vi "I32Notifier Wait2Get.vi"(8 "error in (no error)":errorcluster, 9 "timeout in ms (-1)":i32, 11 "I32Notifier in":refnum<class "I32Notifier.lvclass">) -> (0 "error out":errorcluster, 1 "timed out?":bool, 2 "LastValue":i32, 3 "I32Notifier out":refnum<class "I32Notifier.lvclass">)   [LabVIEW 2018, in "I32Notifier.lvclass"]
uses:
  I32Notifier.lvclass
  I32Notifier.lvclass/I32Notifier.ctl
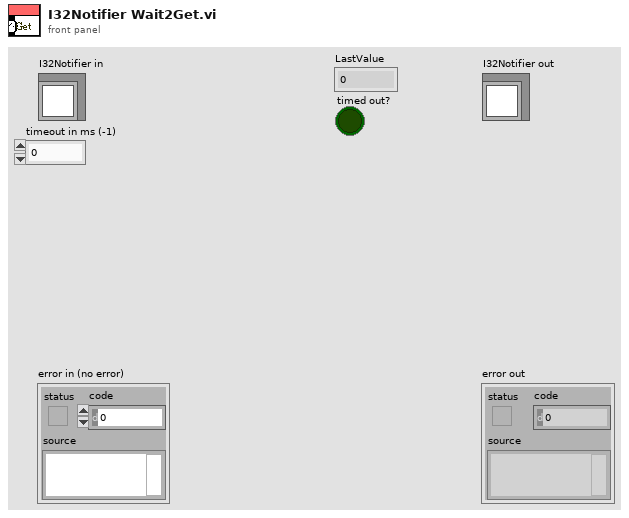
[diagram p1: front panel]
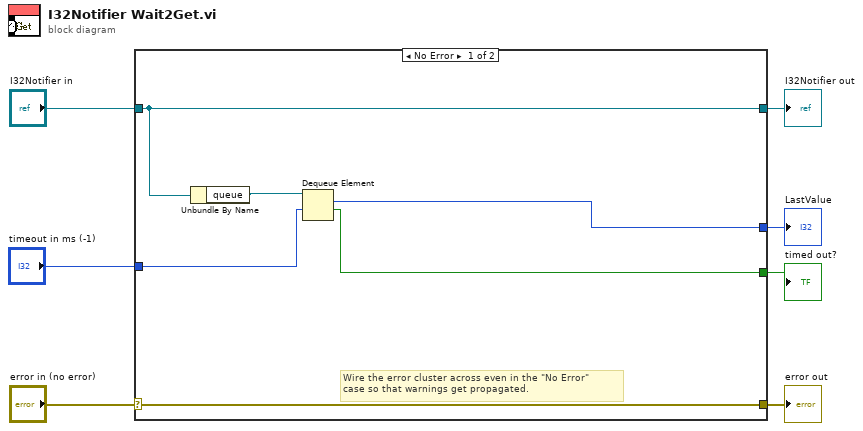
[diagram p0: block diagram]
diagram:
  n1 = case shown="No Error" "error in (no error)" {
    selector: "error in (no error)" -> [w13 w15]
    tunnel: [w13 w15] -> w6
    tunnel: [w12 w14] -> w4
    tunnel: "I32Notifier in" -> [w12 w14]
    tunnel: [w10 _] -> w3
    tunnel: "timeout in ms (-1)" -> [w9 _]
    tunnel: [w8 _] -> w1
    frame No Error {
      # "Wire the error cluster across even in the \"No Error\"\ncase so that warnings get propagated."
      n2 = Unbundle By Name(w12) -> ("queue"=w11:refnum<queue>)
      n3 = Dequeue Element(queue=w11, timeout in ms (-1)=w9) -> (element=w10:i32, timed out?=w8:bool)  [unwired: 1 in, 2 out]
    }
    frame Error {
    }
  }
  "error out" <- w6
  "I32Notifier out" <- w4
  "LastValue" <- w3
  "timed out?" <- w1
